vi "Stop Acquisition.vi"(8 "error in":errorcluster, 11 "Camera Imaqdx in":refnum<class "Camera Imaqdx.lvclass">) -> (0 "error out":errorcluster, 3 "Camera Imaqdx out":refnum<class "Camera Imaqdx.lvclass">)   [LabVIEW 2023, in "Camera.lvlib" / "Camera Imaqdx.lvclass"]
uses:
  Camera Imaqdx.lvclass
  Camera Imaqdx.lvclass/Camera Imaqdx.ctl
  <vilib>/vision/driver/NI_Vision_Acquisition_Software.lvlib
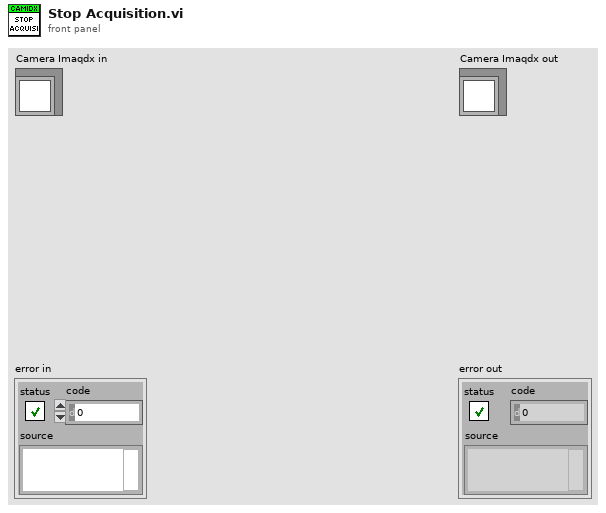
[diagram p1: front panel]
types:
  T1 = typedef "IMAQdx.ctl" = refnum<k21>
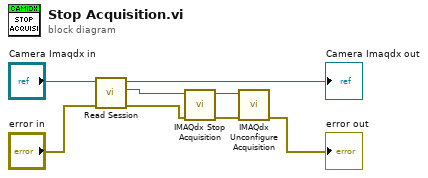
[diagram p0: block diagram]
diagram:
  n1 = call "Read Session.vi"("error in (no error)"="error in", "Camera Imaqdx in"="Camera Imaqdx in") -> ("error out"=w4:errorcluster, "IMAQdx Session"=w1:T1, "Camera Imaqdx out"=→"Camera Imaqdx out":refnum<class "Camera Imaqdx.lvclass">)  [unwired: 7 in]
  n2 = call <vilib>:"IMAQdx Stop Acquisition.vi"("error in"=w4, "Session In"=w1) -> ("error out"=w7:errorcluster, "Session Out"=w5:T1)  [unwired: 8 in]
  n3 = call <vilib>:"IMAQdx Unconfigure Acquisition.vi"("error in"=w7, "Session In"=w5) -> ("error out"=→"error out":errorcluster)  [unwired: 8 in, 1 out]
